vi "Clear Hardware.vi"(2 "error in (no error)":errorcluster, 3 "ArduinoDAC in":refnum<class "ArduinoDAC.lvclass">) -> (0 "error out":errorcluster, 1 "ArduinoDAC out":refnum<class "ArduinoDAC.lvclass">)   [LabVIEW 2013, in "ArduinoDAC.lvclass"]
doc: "This VI resets any necessary hardware so that the device will be ready for the next run."
uses:
  ArduinoDAC.lvclass
  ArduinoDAC.lvclass/ArduinoDAC.ctl
  <vilib>/Instr/_visa.llb/VISA Open Access Mode.ctl
panel:
  out "read buffer":string
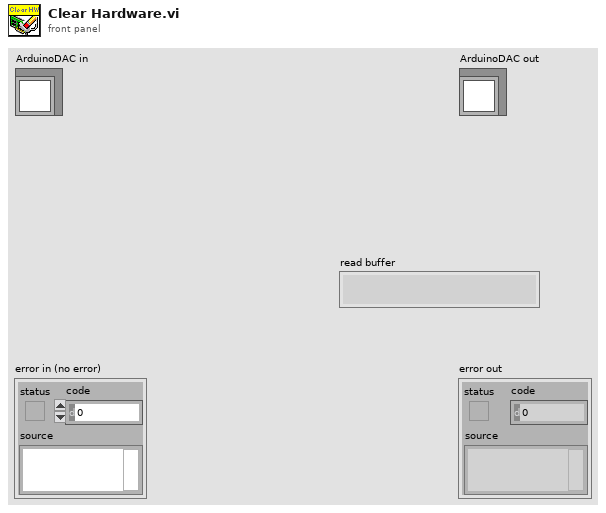
[diagram p1: front panel]
types:
  T1 = typedef "VISA Open Access Mode.ctl" = u32
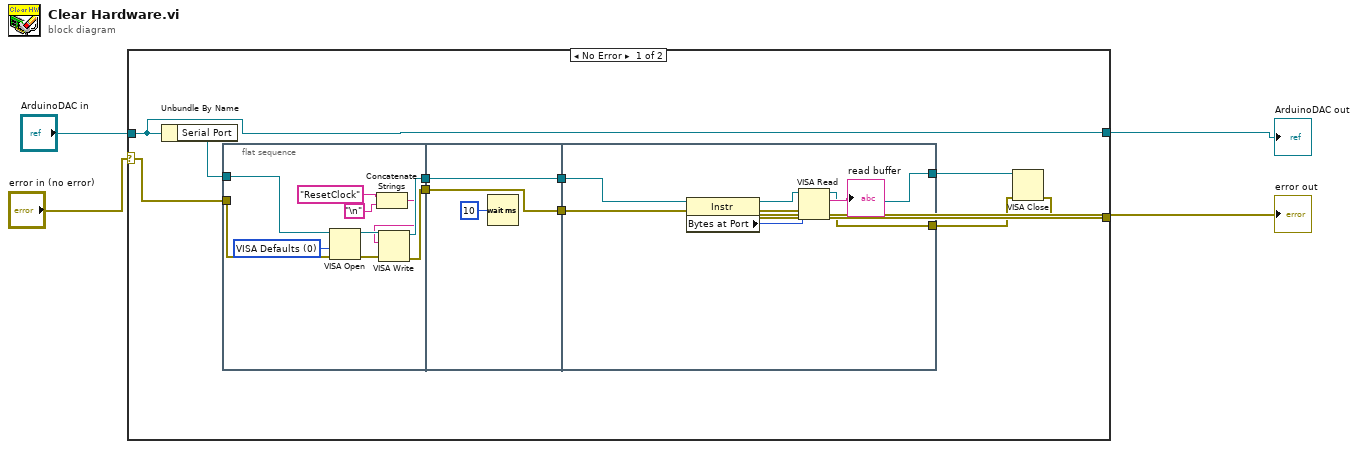
[diagram p0: block diagram]
diagram:
  n1 = case shown="No Error" "error in (no error)" {
    selector: "error in (no error)" -> [w12 w37]
    tunnel: [w11 w37] -> w3
    tunnel: [w14 w36] -> w1
    tunnel: "ArduinoDAC in" -> [w14 w36]
    frame No Error {
      n2 = Unbundle By Name(w14) -> ("Serial Port"=w13:refnum<visa-resource-name>)
      n3 = flat-sequence {
        tunnel: w13 -> [w24]
        tunnel: w12 -> [w23]
        tunnel: [w19] -> w9
        tunnel: [w18] -> w7
        tunnel: [w26] -> w10
        tunnel: w9 -> [w26]
        tunnel: [w25] -> w8
        tunnel: w7 -> [w25]
        tunnel: w10 -> [w31]
        tunnel: w8 -> [w30]
        tunnel: [w29] -> w6
        tunnel: [w28] -> w5
        frame #0 {
          w22 = T1 0 items=["VISA Defaults"=0, "Exclusive Lock"=1, "Load Configured Settings"=4] ("Access Mode")
          n4 = VISA Open(access mode=w22, error in (no error)=w23, VISA resource name=w24) -> (VISA resource name=w21:refnum<visa-resource-name>, error out=w20:errorcluster)  [unwired: 2 in]
          n5 = Concatenate Strings("ResetClock" ("write buffer"), "\n") -> (w15:string)
          n6 = VISA Write(VISA resource name=w21, write buffer=w15, error in (no error)=w20) -> (VISA resource name out=w19:refnum<visa-resource-name>, error out=w18:errorcluster)  [unwired: 1 out]
        }
        frame #1 {
          n7 = Wait (ms)(milliseconds to wait=u32 10) -> ()  [unwired: 1 out]
        }
        frame #2 {
          n8 = property class="Instr"(reference=w31, error in=w30) -> (reference out=w33:refnum<visa-resource-name>, error out=w34:errorcluster, "Bytes at Port"=w35:u32)
          n9 = VISA Read(VISA resource name=w33, byte count=w35, error in (no error)=w34) -> (VISA resource name out=w29:refnum<visa-resource-name>, read buffer=→"read buffer":string, error out=w28:errorcluster)  [unwired: 1 out]
        }
      }
      n10 = VISA Close(VISA resource name=w6, error in (no error)=w5) -> (error out=w11:errorcluster)
    }
    frame Error {
    }
  }
  "error out" <- w3
  "ArduinoDAC out" <- w1
